vi "stage_sim_close.vi"(10 "serial-numbers":string[](array[string]), 11 ".NET Refnum in":refnum<k24>) -> ()   [LabVIEW 2024]
uses:
  O:/DSG/Tyler/EIC/DIRC/daq/automated/Thorlabs.MotionControl.DeviceManagerCLI.dll
  Thorlabs.MotionControl.DeviceManagerCLI.dll
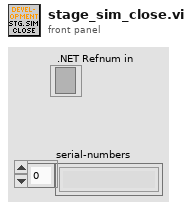
[diagram p1: front panel]
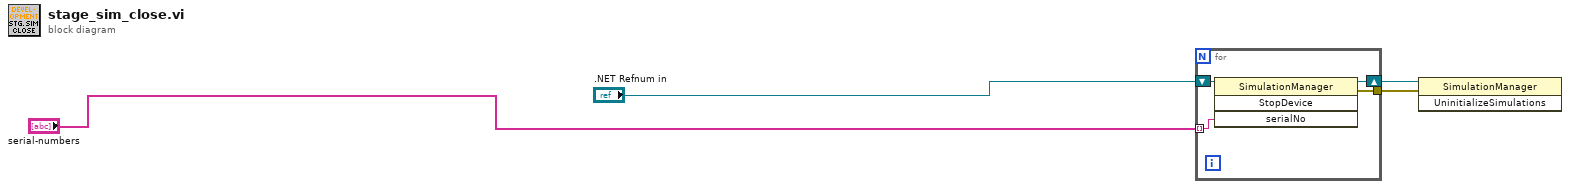
[diagram p0: block diagram]
diagram:
  n1 = for {
    tunnel: [w8] -> w1
    shift-right: [w7] -> w2
    shift-left: ".NET Refnum in" -> [w6]
    tunnel: "serial-numbers" -> [w5] mode=indexing
    n2 = invoke class="SimulationManager" method="StopDevice"(reference=w6, "serialNo"=w5) -> (reference out=w7:refnum<k24>, error out=w8:errorcluster)  [unwired: 2 in, 2 out]
  }
  n3 = invoke class="SimulationManager" method="UninitializeSimulations"(reference=w2, error in=w1) -> ()  [unwired: 1 in, 3 out]
